vi "SetControlEnableSwitch.vi"(6 "?":bool, 8 "error in (no error)":errorcluster, 9 "True Disable":string[](array[string])=["", ""], 10 "True Enable":string[](array[string])=["", ""], 11 "CtlLookup In":T1) -> (0 "error out":errorcluster, 3 "CtlLookup Out":T1)   [LabVIEW 2020, in "CtlReferences_API.lvlib"]
doc: "This VI will Enable/Disable the controls specified by name"
uses:
  CtlReferences_API.lvlib
  TypeDefs/CtlLookup.ctl
  CtlReferences.lvclass
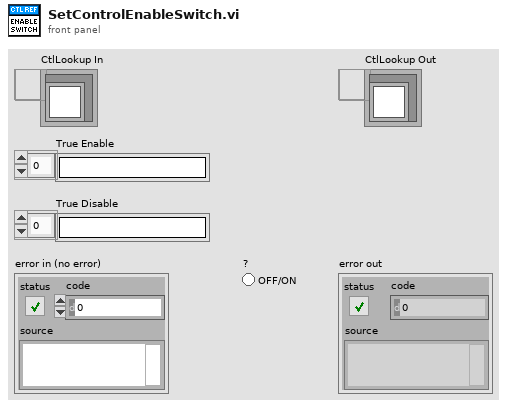
[diagram p1: front panel]
types:
  T1 = typedef "CtlReferences.lvlib/CtlReferences.lvclass/CtlLookup.ctl" = refnum<data-value>
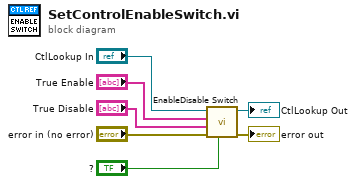
[diagram p0: block diagram]
diagram:
  n1 = call "EnableDisable Switch.vi"("?"="?", "error in (no error)"="error in (no error)", "True Disable"="True Disable", "True Enable"="True Enable", "CtlLookup Out"="CtlLookup In") -> ("error out"=→"error out":errorcluster, "CtlLookup Out"=→"CtlLookup Out":T1)  [unwired: 5 in]
